vi "DHE_close_driver.vi"(0 "fd":i32, 11 "error in (no error)":errorcluster) -> (15 "error out":errorcluster)   [LabVIEW 2016]
doc: "This VI closes the I/O interface with the instrument."
panel:
  out "error_code":i32
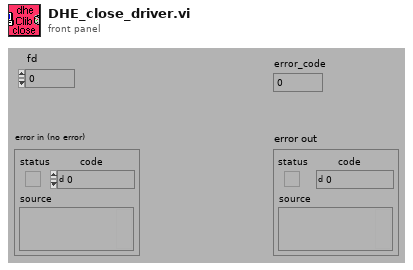
[diagram p1: front panel]
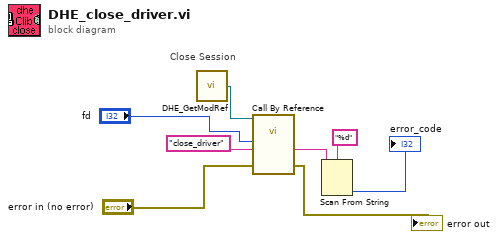
[diagram p0: block diagram]
diagram:
  # "Close Session"
  n1 = call "DHE_GetModRef.vi"() -> ("DHE_ModRef"=w8:refnum<vi>)  [unwired: 9 out]
  n2 = call-by-ref "?"(reference=w8, "error in (no error)"="error in (no error)", "function"="close_driver", "fd in"="fd") -> ("error out"=→"error out":errorcluster, "str result"=w6:string)  [unwired: 6 in, 4 out]
  n3 = Scan From String(format string="%d", input string=w6) -> (output 1=→"error_code":i32)  [unwired: 2 in, 4 out]
